vi "ThreadCfg - Read TxPkt Config.vi"(8 "error in (no error)":errorcluster, 11 "Node Ptr In":T3 format="%.0x") -> (0 "error out":errorcluster, 2 "threadOptions":T1 {"pclDecimation" max=16 step=1; "loopPeriod" min=-2 max=16 step=1; "targetPriority" min=-2 max=16 step=1; "targetProcessor" min=-2 max=16 step=1}, 3 "Node Ptr Out":T3 format="%.0x")   [LabVIEW 2016, in "UDP-Custom-Device System Explorer.lvlib"]
uses:
  UDP-Custom-Device System Explorer.lvlib
  <vilib>/NI Veristand/Custom Device API/Custom Device Item Ref.ctl
  Types/Threading/Thread Configuration.ctl
  Types/Threading/Thread Sync Reference.ctl
  Property Accessors/Tx Packet Accessors.lvlib
  Property Accessors/Shared Packet Accessors.lvlib
  <vilib>/NI VeriStand/Custom Device API/Custom Device API.lvlib
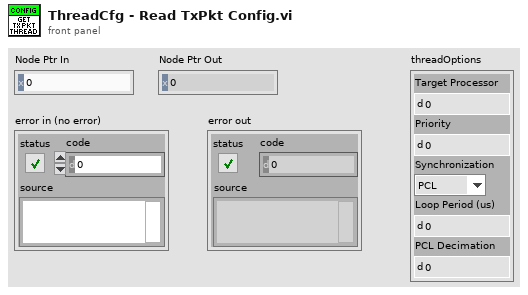
[diagram p1: front panel]
types:
  T1 = typedef "UDP-Custom-Device System Explorer.lvlib/Thread Configuration.ctl" = cluster{"targetProcessor":i8, "targetPriority":i16, "Synchronization":T2, "loopPeriod":i32, "pclDecimation":u16}
  T2 = typedef "UDP-Custom-Device System Explorer.lvlib/Thread Sync Reference.ctl" = enum16{"PCL", "Async"}
  T3 = typedef "Custom Device API.lvlib/Custom Device Item Ref.ctl" = u64
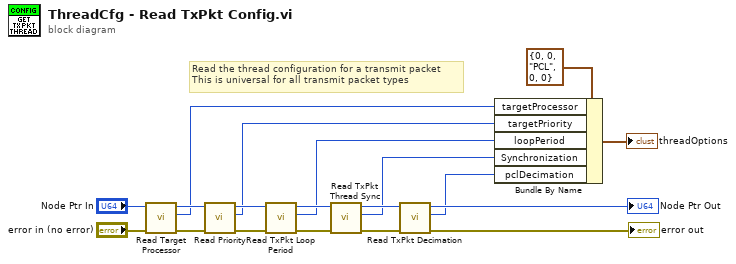
[diagram p0: block diagram]
diagram:
  # "Read the thread configuration for a transmit packet\nThis is universal for all transmit packet types"
  n1 = call "Read Target Processor.vi"("error in (no error)"="error in (no error)", "Node Ptr"="Node Ptr In") -> ("error out"=w16:errorcluster, "targetProcessor"=w1:i8, "Node Ptr out"=w17:T3)  [unwired: 7 in]
  n2 = call "Read Priority.vi"("error in (no error)"=w16, "Node Ptr"=w17) -> ("error out"=w14:errorcluster, "targetPriority"=w2:i16, "Node Ptr out"=w15:T3)  [unwired: 7 in]
  n3 = call "Read TxPkt Loop Period.vi"("error in (no error)"=w14, "Node Ptr"=w15) -> ("error out"=w13:errorcluster, "loopPeriod"=w3:i32, "Node Ptr out"=w12:T3)  [unwired: 7 in]
  n4 = call "Read TxPkt Thread Sync.vi"("error in (no error)"=w13, "Node Ptr"=w12) -> ("error out"=w10:errorcluster, "threadSync"=w4:T2, "Node Ptr out"=w11:T3)  [unwired: 7 in]
  n5 = call "Read TxPkt Decimation.vi"("error in (no error)"=w10, "Node Ptr"=w11) -> ("error out"=→"error out":errorcluster, "Decimation"=w5:u16, "Node Ptr out"=→"Node Ptr Out":T3)  [unwired: 7 in]
  n6 = Bundle By Name(cluster=T1 {"targetProcessor"=0, "targetPriority"=0, "Synchronization"=enum."PCL", "loopPeriod"=0, "pclDecimation"=0} ("threadOptions"), "targetProcessor"=w1, "targetPriority"=w2, "loopPeriod"=w3, "Synchronization"=w4, "pclDecimation"=w5) -> (→"threadOptions":T1)
